vi "pid.vi"(0 "kp":dbl, 1 "err":dbl, 5 "kd":dbl, 7 "ki":dbl, 9 "dt":dbl, 11 "intergral":dbl, 12 "old_err":dbl) -> (4 "curr_err":dbl, 6 "curr_integral":dbl, 8 "y":dbl)   [LabVIEW 2019]
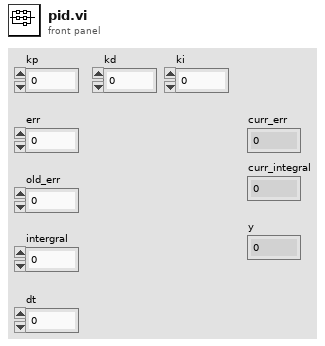
[diagram p1: front panel]
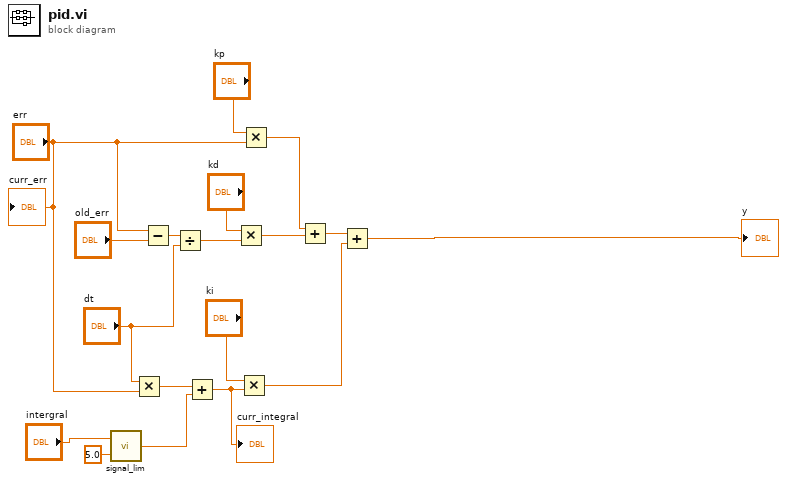
[diagram p0: block diagram]
diagram:
  n1 = call "signal_lim.vi"("lim"=5.0, "x"="intergral") -> ("y"=w2:dbl)
  n2 = Multiply(x="dt", y="err") -> (x*y=w15:dbl)
  n3 = Subtract(x="err", y="old_err") -> (x-y=w14:dbl)
  n4 = Divide(x=w14, y="dt") -> (x/y=w12:dbl)
  n5 = Add(x=w15, y=w2) -> (x+y=w9:dbl)
  "curr_integral" <- w9
  n6 = Multiply(x="kd", y=w12) -> (x*y=w8:dbl)
  n7 = Multiply(x="ki", y=w9) -> (x*y=w5:dbl)
  n8 = Multiply(x="kp", y="err") -> (x*y=w7:dbl)
  n9 = Add(x=w7, y=w8) -> (x+y=w6:dbl)
  n10 = Add(x=w6, y=w5) -> (x+y=→"y":dbl)
  "curr_err" <- "err"
